vi "Create FP Item.vi"(6 "Cluster Component":bool, 8 "error in (no error)":errorcluster, 10 "GObject In":refnum<vi>, 11 "GSelect in":refnum<class "Select.lvclass">) -> (0 "error out":errorcluster, 1 "Is Control":bool, 2 "Is Indicator":bool, 3 "GSelect out":refnum<class "Select.lvclass">, 4 "All Objects Created":refnum<class "Object.lvclass">[](array[class]), 5 "Is Visible":bool)   [LabVIEW 2017, in "Front Panel Publisher.lvlib" / "Select.lvclass"]
uses:
  Select.lvclass
  Control_class/Control.lvclass
  Object_class/Object.lvclass
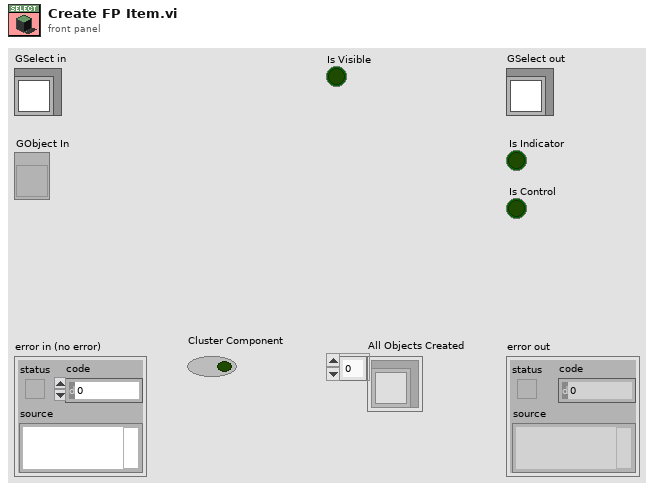
[diagram p1: front panel]
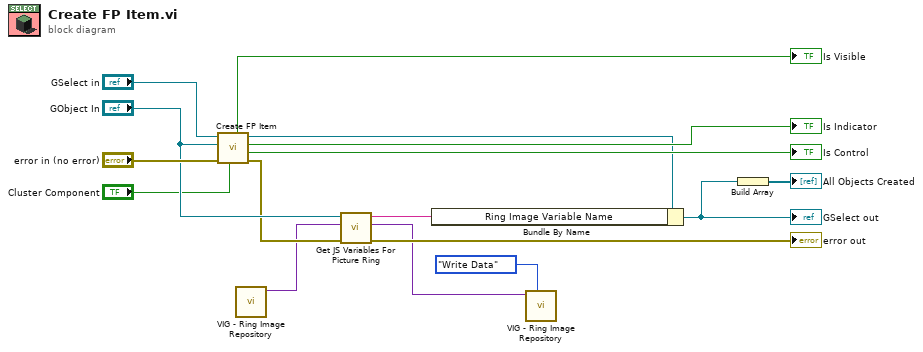
[diagram p0: block diagram]
diagram:
  n1 = call-parent "Create FP Item.vi"("Cluster Component"="Cluster Component", "error in (no error)"="error in (no error)", "GObject In"="GObject In", "GControl in"="GSelect in") -> ("error out"=w9:errorcluster, "Is Control"=→"Is Control":bool, "Is Indicator"=→"Is Indicator":bool, "GControl out"=w7:refnum<class "Select.lvclass">, "Is Visible"=→"Is Visible":bool)  [unwired: 2 in, 1 out]
  n2 = call "VIG - Ring Image Repository.vi"() -> ("Variant Data Out"=w6:variant)  [unwired: 10 in, 1 out]
  n3 = call "Get JS Variables For Picture Ring.vi"("error in (no error)"=w9, "Ring Images In"=w6, "Ring in"="GObject In") -> ("error out"=→"error out":errorcluster, "Ring Images Out"=w5:variant, "Ring Image Variable Name"=w11:string)  [unwired: 6 in]
  n4 = Bundle By Name(cluster=w7, "Ring Image Variable Name"=w11) -> (w3:refnum<class "Select.lvclass">)
  "GSelect out" <- w3
  n5 = call "VIG - Ring Image Repository.vi"("Method (Read)"=enum16{"Read Data", "Write Data"}."Write Data", "Variant Data In"=w5) -> ()  [unwired: 8 in, 2 out]
  n6 = Build Array(w3) -> (→"All Objects Created":refnum<class "Select.lvclass">[])
